vi "Create.vi"   [LabVIEW 2018, in "Toolkit.lvlib" / "Listener.lvclass"]
doc: "Creates a new Listener object and allocates memory within the libssh2lv shared library for a corresponding Listener struct."
uses:
  Listener.lvclass
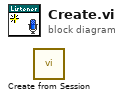
[diagram p0: block diagram]
diagram:
  n1 = call "Create from Session.vi"() -> ()  [unwired: 10 in, 2 out]
